vi "생산자소비자(이벤트).vi"() -> ()   [LabVIEW 2014]
uses:
  <vilib>/Analysis/NI_AALBase.lvlib
panel:
  in  "기다림":i32
  out "웨이브폼 그래프":dbl[](graph)
  in  "정지":bool
  in  "확인 버튼":bool
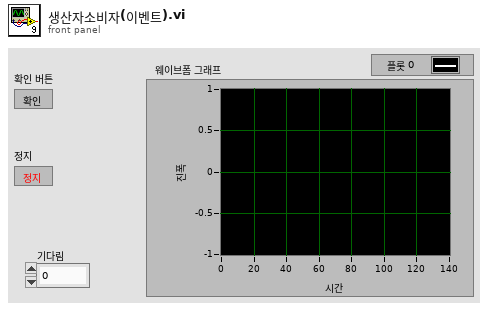
[diagram p1: front panel]
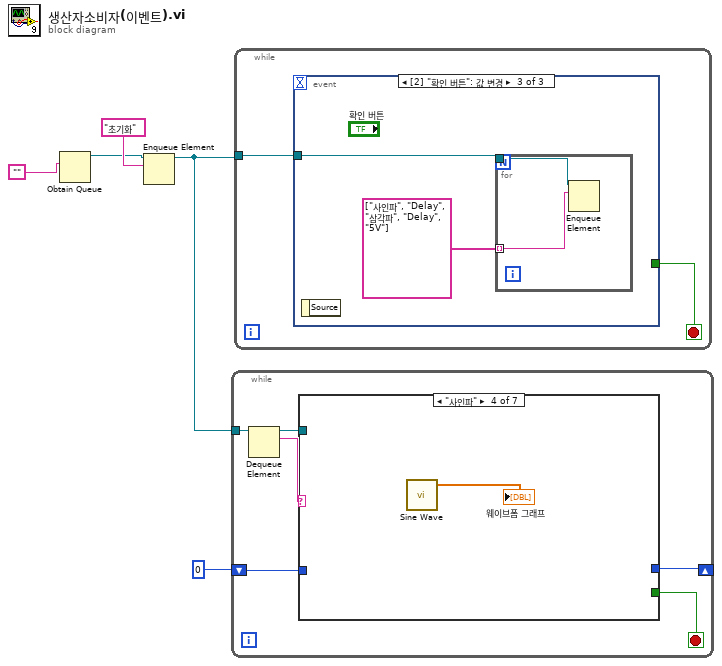
[diagram p0: block diagram]
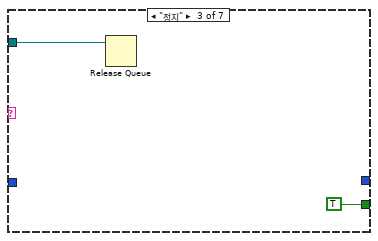
[diagram p4: hidden frame]
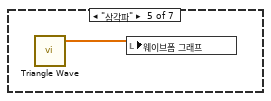
[diagram p5: hidden frame]
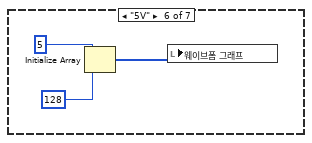
[diagram p6: hidden frame]
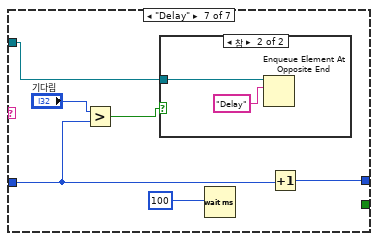
[diagram p7: hidden frame]
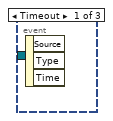
[diagram p9: hidden frame]
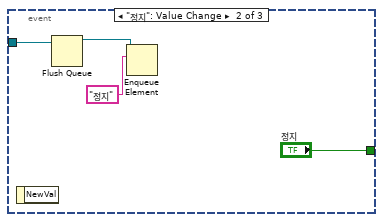
[diagram p10: hidden frame]
diagram:
  n1 = Obtain Queue(element data type="") -> (queue out=w1:refnum<queue>)  [unwired: 4 in, 2 out]
  n2 = Enqueue Element(queue=w1, element="초기화") -> (queue out=w3:refnum<queue>)  [unwired: 2 in, 2 out]
  n3 = while {
    shift-right: [w6] -> _
    shift-left: 0 -> [w7]
    tunnel: w3 -> [w9]
    stop <- w8 stop-if-true
    n4 = Dequeue Element(queue=w9) -> (queue out=w11:refnum<queue>, element=w10:string)  [unwired: 2 in, 2 out]
    n5 = case shown="\"사인파\"" w10 {
      tunnel: w11 -> [_ _ w13 _ _ _ w22]
      tunnel: [_ _ TRUE _ _ _ _] -> w8
      tunnel: w7 -> [_ _ _ _ _ _ w20]
      tunnel: [_ _ _ _ _ _ w19] -> w6
      frame Default {
      }
      frame "초기화" {
      }
      frame "정지" {
        n6 = Release Queue(queue=w13) -> ()  [unwired: 2 in, 3 out]
      }
      frame "사인파" {
        n7 = call <vilib>:"Sine Wave.vi"() -> ("sine wave"=→"웨이브폼 그래프":dbl[])  [unwired: 5 in, 2 out]
      }
      frame "삼각파" {
        n8 = call <vilib>:"Triangle Wave.vi"() -> ("triangle wave"=w15:dbl[])  [unwired: 5 in, 2 out]
        n9 = local write "웨이브폼 그래프"(w15) -> ()
      }
      frame "5V" {
        n10 = Initialize Array(5, 128) -> (w16:i32[])
        n11 = local write "웨이브폼 그래프"(w16) -> ()
      }
      frame "Delay" {
        n12 = Greater?(x="기다림", y=w20) -> (0:w23:bool)
        n13 = case shown="참" w23 {
          tunnel: w22 -> [_ w26]
          frame False {
          }
          frame True {
            n14 = Enqueue Element At Opposite End(queue=w26, element="Delay") -> ()  [unwired: 2 in, 3 out]
          }
        }
        n15 = Wait (ms)(milliseconds to wait=100) -> ()  [unwired: 1 out]
        n16 = Increment(x=w20) -> (x+1=w19:i32)
      }
    }
  }
  n17 = while {
    tunnel: w3 -> [w27]
    stop <- w28 stop-if-true
    n18 = event shown="[2] \"확인 버튼\": 값 변경" {
      selector: _ -> [_ _ _]
      dyn-events: _ -> [_ _ _]
      timeout: _ -> [_ _ _]
      tunnel: [_ "정지" _] -> w28
      tunnel: w27 -> [_ w30 w34]
      event Timeout {
        n19 = event-data() -> ()  [unwired: 1 in, 3 out]
      }
      event "정지": Value Change {
        n20 = event-data() -> ()  [unwired: 1 in, 1 out]
        n21 = Flush Queue(queue=w30) -> (queue out=w29:refnum<queue>)  [unwired: 1 in, 2 out]
        n22 = Enqueue Element(queue=w29, element="정지") -> ()  [unwired: 2 in, 3 out]
      }
      event "확인 버튼": Value Change {
        n23 = event-data() -> ()  [unwired: 1 in, 1 out]
        n24 = for {
          tunnel: w34 -> [w36]
          tunnel: string[] ["사인파", "Delay", "삼각파", "Delay", "5V"] -> [w35] mode=indexing
          n25 = Enqueue Element(queue=w36, element=w35) -> ()  [unwired: 2 in, 3 out]
        }
      }
    }
  }
